vi "Teleop.vi"(10 "Match Info":T2={"Autonomous Elapsed Seconds"=0.0, "TeleOp Elapsed Seconds"=34.379, "Disabled Elapsed Seconds"=12.859, "Visited Autonomous"=FALSE, "Visited TeleOp"=TRUE, "Visited Disabled"=TRUE, "Autonomous Settings"={"Autonomous Style"=enum."Independent", "VI Refnum"=refnum}}, 11 "Call Context":T3=enum."Execute") -> ()   [LabVIEW 2015]
doc: "This VI is called for each TeleOp packet received from the DS where the robot is not disabled. It is often used to read from the joysticks and update I/O or to update setpoints for timed control loops. It should complete and return within 20 milliseconds or it may miss DS packets."
uses:
  <vilib>/Rock Robotics/WPI/DriverStation/WPI_DriverStationDerivedRobotMode.ctl
  <vilib>/Rock Robotics/WPI/DriverStation/WPI_DriverStationMatch Info.ctl
  MotorSpeedState.ctl
  <vilib>/Rock Robotics/WPI/Utilities/WPI_GetSetVariantRefNum.vi
  <vilib>/Rock Robotics/Network Tables/SD Write Numeric Array.vi
  <vilib>/Rock Robotics/Network Tables/SD Write Boolean Array.vi
  <vilib>/Rock Robotics/Network Tables/SD Read Boolean.vi
  <vilib>/Rock Robotics/Network Tables/SD Read Number.vi
  <vilib>/Rock Robotics/Network Tables/NT Write Boolean.vi
panel:
  out "Motor output Plot":cluster{"Applied Throttle":dbl}(graph)={"Applied Throttle"=-0.0019550342130987292}
  out "Position Closed Loop Plots":cluster{dbl, "Sensor Velocity":dbl}(graph)={-0.002210038162407613, "Sensor Velocity"=-0.00341796875}
  in  "Ramp Rate":dbl=0.4
  in  "D":dbl=10.0
  in  "I":dbl=0.0001
  in  "P":dbl=0.4
  in  "Drive Train Scale":dbl(slide)=0.7857142857142857 scale=0.0..1.0
  in  "Scale: Dan's Hand":dbl(slide)=0.354978354978355 scale=0.0..1.0
  out "Total Current (Arm)":dbl(graph)
  out "Total Current (Arm + Drive Train)":dbl(graph)
  out "all currents (A)":dbl[](array[numeric])
  out "current (A)":dbl
  out "Total Current (Arm + Drive Train)":dbl
  out "Individual Currents":T1(graph)
  in  "Arm Scale":dbl(slide)=0.1 scale=0.0..0.6
  out "Sample Slider 0":dbl(slide) scale=0.0..5.0
  out "Sample Boolean 1":bool
  out "Sample Boolean 0":bool
  # "A-0\nB-1\nX-2\nY-3\nLB-4\nRB-5"
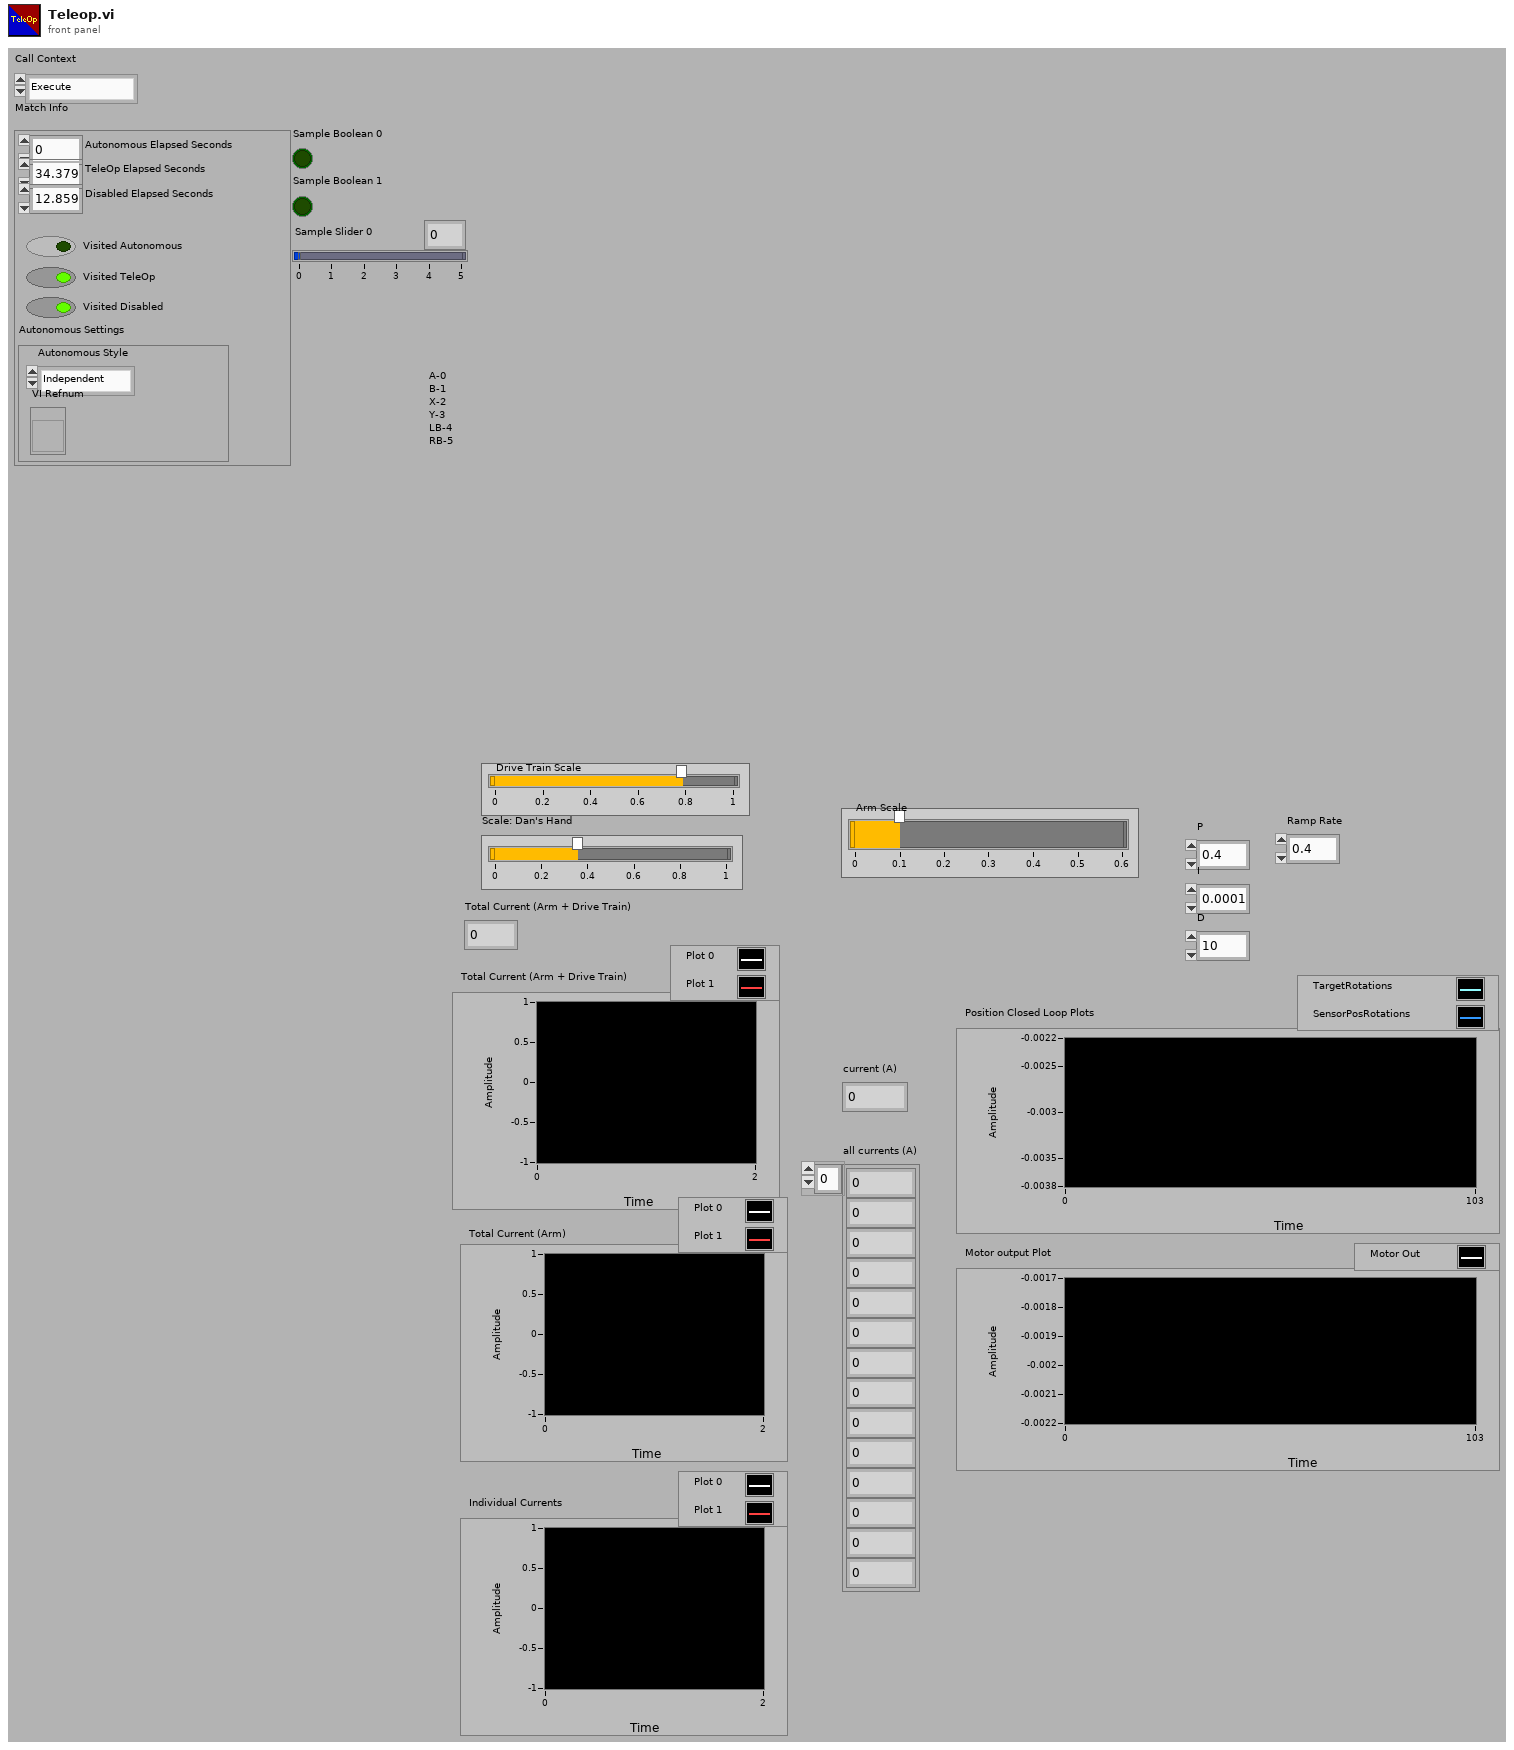
[diagram p1: front panel]
types:
  T1 = cluster{"Current":dbl, "Current":dbl, "Current":dbl, "Current":dbl, "Current":dbl}
  T2 = typedef "WPI_DriverStationMatch Info.ctl" = cluster{"Autonomous Elapsed Seconds":dbl, "TeleOp Elapsed Seconds":dbl, "Disabled Elapsed Seconds":dbl, "Visited Autonomous":bool, "Visited TeleOp":bool, "Visited Disabled":bool, "Autonomous Settings":cluster{"Autonomous Style":enum16{"Iterative", "Independent"}, "VI Refnum":refnum<vi>}}
  T3 = typedef "WPI_DriverStationDerivedRobotMode.ctl" = enum16{"Init", "Execute", "Stop"}
  T4 = typedef "MotorSpeedState.ctl" = enum16{"Half-speed", "Full-speed"}
  T5 = typedef "WPI_JoystickDevRef.ctl" = cluster{"Device":T6}
  T6 = typedef "WPI_JoystickDeviceEnum.ctl" = enum16{"USB 0", "USB 1", "USB 2", "USB 3", "USB 4", "USB 5"}
  T7 = typedef "WPI_MotorControlDeviceRef.ctl" = cluster{"DeviceStatus":errorcluster, "Type":T8, "PWM":cluster{"PWM Channel":T9, "DeadBand":T10}, "CAN":cluster{"Device Number":u8, "Control Mode":T11, "Semaphore":T12, "Max Vout":dbl, "TalonSRX Control Mode":T13}, "Invert":bool}
  T8 = typedef "WPI_MotorControlType.ctl" = enum16{"PWM", "CAN", "CANTalonSRX"}
  T9 = typedef "FPGA_DIOPWMChannel.ctl" = enum8{"PWM 0", "PWM 1", "PWM 2", "PWM 3", "PWM 4", "PWM 5", "PWM 6", "PWM 7", "PWM 8", "PWM 9", "PWM MXP 0", "PWM MXP 1", "PWM MXP 2", "PWM MXP 3", "PWM MXP 4", "PWM MXP 5", "PWM MXP 6", "PWM MXP 7", "PWM MXP 8", "PWM MXP 9", "Invalid"}
  T10 = typedef "WPI_PWMDeadband.ctl" = cluster{"Name":string, "maxPositivePwm":i32, "minPositivePwm":i32, "centerPwm":i32, "maxNegativePwm":i32, "minNegativePwm":i32, "angularRange":u16}
  T11 = typedef "WPI_CANJaguar_ControlMode.ctl" = enum8{"Percent VBus", "Current", "Speed", "Position", "Voltage"}
  T12 = typedef "Semaphore RefNum" = refnum<k1>
  T13 = typedef "WPI_CANTalonSRX_APIControlMode.ctl" = enum8{"Percent VBus", "Speed", "Position", "Slave", "Unchanged / Invalid", "Voltage Compensation", "Current", "Motion Profile"}
  T14 = typedef "WPI_CANTalonSRX_GlobalStatus.ctl" = cluster{"Applied Throttle":dbl, "Module Enabled":bool, "CAN Error":errorcluster, "Closed Loop Error":dbl, "Forward Limit Switch Closed":bool, "Reverse Limit Switch Closed":bool, "Sensor Position":dbl, "Sensor Velocity":dbl, "Current":dbl, "Sticky Fault - Over Temp":bool, "Sticky Fault - Under Voltage":bool, "Sticky Fault - Forward Limit":bool, "Sticky Fault - Reverse Limit":bool, "Sticky Fault - Forward Soft Limit":bool, "Sticky Fault - Reverse Soft Limit":bool, "Brake is Enabled":bool, "Encoder Position":dbl, "Encoder Velocity":dbl, "Encoder Index Count":dbl, "Encoder A Pin State":bool, "Encoder B Pin State":bool, "Encoder Index Pin State":bool, "Analog In":dbl, "Analog In Velocity":dbl, "Temperature (C)":dbl, "Battery Voltage":dbl, "Control 5 Is Supported":bool, "Current Profile Slot Select":dbl, "Pos Div 8":bool, "Vel Div 4":bool, "Pulse Width Position":i32, "Pulse Width Velocity":i32, "Pulse Width Rise To Rise (us)":i32, "Pulse Width Rise To Fall (us)":i32, "Mot Prof Active Is Under Run":bool, "Mot Prof Active Has Under Run":bool, "Mot Prof Active Is Last":bool, "Mot Prof Active Velocity Only":bool, "Mot Prof Active Is Valid":bool, "Mot Prof Buffer Is Full":bool, "Mot Prof Active Profile Slot Select":i32, "Mot Prof NextID":i32, "Mot Prof Count":i32, "Mot Prof Active Velocity":dbl, "Mot Prof Active Position":dbl, "Mot Prof Output Enable":i32}
  T15 = typedef "WPI_RobotDriveDevRef.ctl" = cluster{"DevStatus":errorcluster, "Motors[]":T7[], "Square Inputs":bool, "Max Output":dbl}
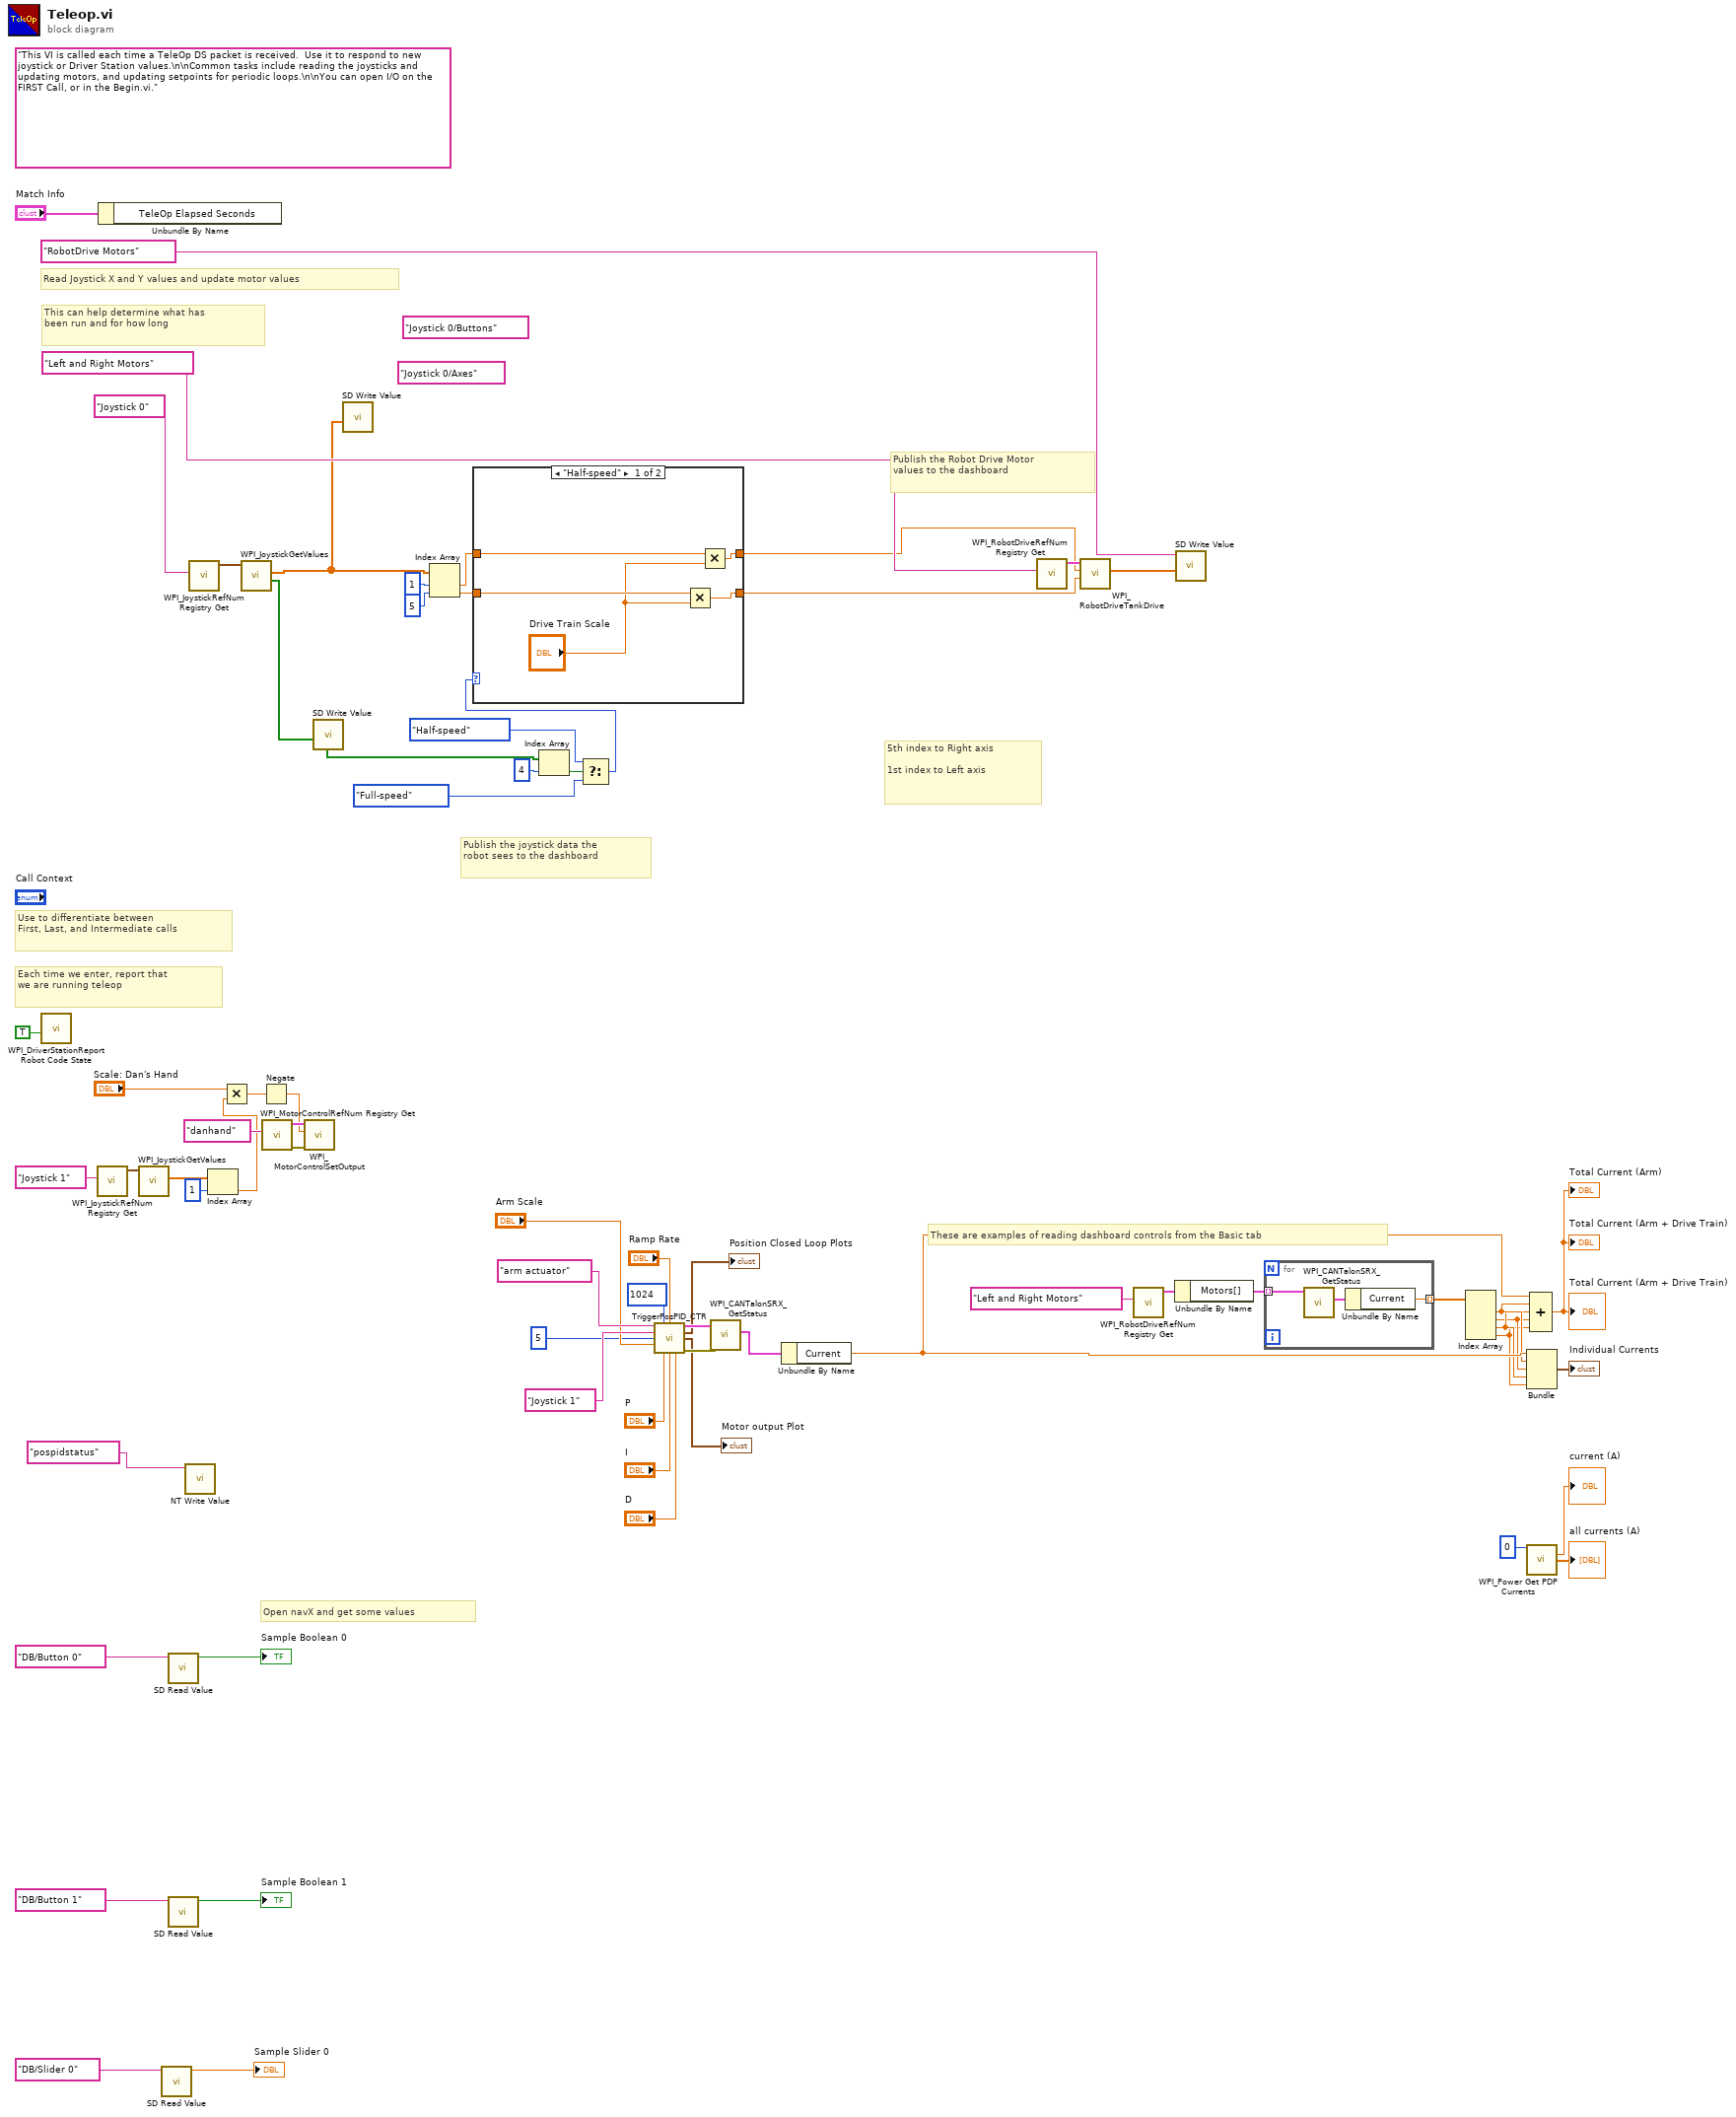
[diagram p0: block diagram]
diagram:
  (unwired) "Joystick 0/Axes" ("Name")
  (unwired) "Joystick 0/Buttons" ("Name")
  (unwired) "This VI is called each time a TeleOp DS packet is received.  Use it to respond to new joystick or Driver Station values.\n\nCommon tasks include reading the joysticks and updating motors, and updating setpoints for periodic loops.\n\nYou can open I/O on the FIRST Call, or in the Begin.vi."
  # "5th index to Right axis\n\n1st index to Left axis"
  # "Open navX and get some values"
  # "These are examples of reading dashboard controls from the Basic tab"
  # "Publish the Robot Drive Motor\nvalues to the dashboard"
  # "Publish the joystick data the\nrobot sees to the dashboard"
  # "Each time we enter, report that\nwe are running teleop"
  # "Use to differentiate between\nFirst, Last, and Intermediate calls"
  # "This can help determine what has\nbeen run and for how long"
  # "Read Joystick X and Y values and update motor values"
  n1 = call <vilib>:"WPI_DriverStationReport Robot Code State.vi"("TeleOp"=TRUE ("Autonomous")) -> ()  [unwired: 10 in, 1 out]
  n2 = call <vilib>:"WPI_JoystickRefNum Registry Get.vi"("refnum name"="Joystick 1") -> ("JoystickDevRef"=w50:T5)  [unwired: 1 in, 9 out]
  n3 = Unbundle By Name("Match Info") -> ()  [unwired: 1 out]
  n4 = call <vilib>:"WPI_JoystickGetValues.vi"("JoystickDevRef"=w50) -> ("Axes"=w48:dbl[])  [unwired: 6 in, 4 out]
  n5 = call-poly <vilib>:"SD Read Value.vi"("Name"="DB/Slider 0" ("refnum name")) -> ("Numeric"=→"Sample Slider 0":dbl)  [unwired: 8 in, 2 out]
  n6 = call-poly <vilib>:"SD Read Value.vi"("Name"="DB/Button 0" ("refnum name")) -> ("Boolean"=→"Sample Boolean 0":bool)  [unwired: 8 in, 2 out]
  n7 = call-poly <vilib>:"SD Read Value.vi"("Name"="DB/Button 1" ("refnum name")) -> ("Boolean"=→"Sample Boolean 1":bool)  [unwired: 8 in, 2 out]
  n8 = call-poly <vilib>:"NT Write Value.vi"("Name"="pospidstatus") -> ()  [unwired: 10 in, 1 out]
  n9 = call <vilib>:"WPI_JoystickRefNum Registry Get.vi"("refnum name"="Joystick 0") -> ("JoystickDevRef"=w63:T5)  [unwired: 1 in, 9 out]
  n10 = Index Array(array=w48, index=1) -> (element=w19:dbl)
  n11 = Multiply(x="Scale: Dan's Hand", y=w19) -> (x*y=w29:dbl)
  n12 = call <vilib>:"WPI_JoystickGetValues.vi"("JoystickDevRef"=w63) -> ("Buttons"=w25:bool[], "Axes"=w51:dbl[])  [unwired: 6 in, 3 out]
  n13 = Negate(x=w29) -> (-x=w17:dbl)
  n14 = call <vilib>:"WPI_MotorControlRefNum Registry Get.vi"("refnum name"="danhand") -> ("error out"=w45:errorcluster, "MotorControlDevRef"=w46:T7)  [unwired: 9 in]
  n15 = call <vilib>:"WPI_MotorControlSetOutput.vi"("error in (no error)"=w45, "Output"=w17, "MotorControlDevRef"=w46) -> ()  [unwired: 6 in, 3 out]
  n16 = call-poly <vilib>:"SD Write Value.vi"("Boolean Array"=w25) -> ()  [unwired: 9 in, 2 out]
  n17 = call-poly <vilib>:"SD Write Value.vi"("Numeric Array"=w51) -> ()  [unwired: 9 in, 2 out]
  n18 = Index Array(array=w51, index #1=1 ("index"), index #2=5 ("index")) -> (element #1=w20:dbl, element #2=w22:dbl)
  n19 = Index Array(array=w25, index=4) -> (element=w26:bool)
  n20 = Select(t=MotorSpeedState."Half-speed", s=w26, f=MotorSpeedState."Full-speed") -> (s? t:f=w24:T4)
  n21 = case shown="\"Half-speed\"" w24 {
    tunnel: [w69 w74] -> w23
    tunnel: w22 -> [w72 w74]
    tunnel: [w70 w73] -> w21
    tunnel: w20 -> [w71 w73]
    frame "Half-speed" {
      n22 = Multiply(x=w72, y="Drive Train Scale") -> (x*y=w69:dbl)
      n23 = Multiply(x=w71, y="Drive Train Scale") -> (x*y=w70:dbl)
    }
    frame "Full-speed", Default {
      # "5th index to Right axis\n\n1st index to Left axis"
    }
  }
  n24 = call "TriggerPosPID_CTR.vi"("Motor Ref Num"="arm actuator" ("refnum name"), "Number Encoder Lines\n(Counts Per Rotation)"=u32 1024 ("Number Encoder Lines\n(Counts Per Rotation)"), "Ramp Rate"="Ramp Rate", "Joystick Refnum"="Joystick 1" ("refnum name"), "arm index"=5 ("index"), "Arm Scale"="Arm Scale", "P"="P", "I"="I", "D"="D") -> ("CAN Talon SRX Ref"=w5:T7, "Position Closed Loop Plots"=→"Position Closed Loop Plots":cluster{dbl, "Sensor Velocity":dbl}, "Motor output Plot"=→"Motor output Plot":cluster{"Applied Throttle":dbl}, "error out"=w4:errorcluster)  [unwired: 3 in]
  n25 = call <vilib>:"WPI_CANTalonSRX_GetStatus.vi"("error in (no error)"=w4, "CAN Talon SRX Ref"=w5) -> ("Talon SRX Status"=w44:T14)  [unwired: 7 in, 2 out]
  n26 = Unbundle By Name(w44) -> ("Current"=w38:dbl)
  n27 = call <vilib>:"WPI_RobotDriveRefNum Registry Get.vi"("refnum name"="Left and Right Motors") -> ("RobotDriveDevRef"=w65:T15)  [unwired: 1 in, 9 out]
  n28 = call <vilib>:"WPI_RobotDriveTankDrive.vi"("Right axis value"=w23, "Left axis value"=w21, "RobotDriveDevRef"=w65) -> ("Motor Values"=w54:dbl[])  [unwired: 6 in, 2 out]
  n29 = call <vilib>:"WPI_RobotDriveRefNum Registry Get.vi"("refnum name"="Left and Right Motors") -> ("RobotDriveDevRef"=w42:T15)  [unwired: 1 in, 9 out]
  n30 = Unbundle By Name(w42) -> ("Motors[]"=w41:T7[])
  n31 = call-poly <vilib>:"SD Write Value.vi"("Numeric Array"=w54, "Name"="RobotDrive Motors") -> ()  [unwired: 8 in, 2 out]
  n32 = for {
    tunnel: w41 -> [w77] mode=indexing
    tunnel: [w75] -> w40 mode=indexing
    n33 = call <vilib>:"WPI_CANTalonSRX_GetStatus.vi"("CAN Talon SRX Ref"=w77) -> ("Talon SRX Status"=w76:T14)  [unwired: 8 in, 2 out]
    n34 = Unbundle By Name(w76) -> ("Current"=w75:dbl)
  }
  n35 = Index Array(array=w40) -> (element #1=w37:dbl, element #2=w35:dbl, element #3=w36:dbl, element #4=w34:dbl)  [unwired: 4 in]
  n36 = Bundle("Current"=w38, "Current"=w37, "Current"=w35, "Current"=w36, "Current"=w34) -> (→"Individual Currents":T1)  [unwired: 1 in]
  n37 = call <vilib>:"WPI_Power Get PDP Currents.vi"("Power Distribution Panel (0)"=u8 0) -> ("current (A)"=→"current (A)":dbl, "all currents (A)"=→"all currents (A)":dbl[])  [unwired: 12 in, 1 out]
  n38 = Compound Arithmetic op=ADD(w38, w37, w36, w35, w34) -> (→"Total Current (Arm + Drive Train)" →"Total Current (Arm + Drive Train)" →"Total Current (Arm)":dbl)
